vi "Orient Curves.vi"(8 "error in (no error)":errorcluster, 9 "Curve 2 In":cluster{"X":dbl, "Y":dbl}[](array[cluster]), 10 "Curve 1 In":cluster{"X":dbl, "Y":dbl}[](array[cluster]), 11 "Tool Funnel in":refnum<class "Tool Funnel.lvclass">) -> (0 "error out":errorcluster, 1 "Curve 2 Out":cluster{"X":dbl, "Y":dbl}[](array[cluster]), 2 "Curve 1 Out":cluster{"X":dbl, "Y":dbl}[](array[cluster]), 3 "Tool Funnel out":refnum<class "Tool Funnel.lvclass">)   [LabVIEW 2019, in "Tool Funnel.lvclass"]
uses:
  Tool Funnel.lvclass
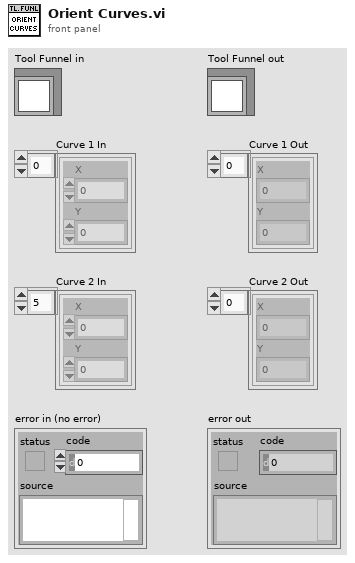
[diagram p1: front panel]
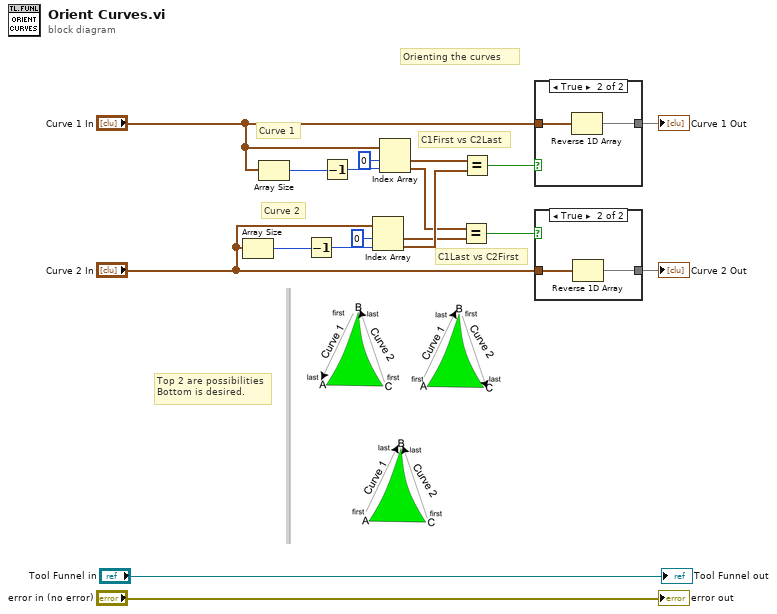
[diagram p0: block diagram]
diagram:
  # "Top 2 are possibilities\nBottom is desired."
  # "C1Last vs C2First"
  # "C1First vs C2Last"
  # "Orienting the curves"
  # "Curve 2"
  # "Curve 1"
  n1 = Array Size(array="Curve 2 In") -> (size(s)=w16:i32)
  n2 = Array Size(array="Curve 1 In") -> (size(s)=w12:i32)
  n3 = Decrement(x=w16) -> (x-1=w14:i32)
  n4 = Decrement(x=w12) -> (x-1=w11:i32)
  n5 = Index Array(array="Curve 2 In", index #1=0 ("index"), index #2=w14) -> (element #1=w6:cluster{"X":dbl, "Y":dbl}, element #2=w7:cluster{"X":dbl, "Y":dbl})
  n6 = Index Array(array="Curve 1 In", index #1=0 ("index"), index #2=w11) -> (element #1=w10:cluster{"X":dbl, "Y":dbl}, element #2=w5:cluster{"X":dbl, "Y":dbl})
  n7 = Equal?(x=w5, y=w6) -> (x = y?=w8:bool)
  n8 = Equal?(x=w10, y=w7) -> (x = y?=w9:bool)
  n9 = case shown="True" w9 {
    tunnel: "Curve 1 In" -> [w19 w21]
    tunnel: [w19 w20] -> w2
    frame False {
    }
    frame True {
      n10 = Reverse 1D Array(array=w21) -> (reversed array=w20:cluster{"X":dbl, "Y":dbl}[])
    }
  }
  "Curve 1 Out" <- w2
  n11 = case shown="True" w8 {
    tunnel: "Curve 2 In" -> [w22 w24]
    tunnel: [w22 w23] -> w3
    frame False {
    }
    frame True {
      n12 = Reverse 1D Array(array=w24) -> (reversed array=w23:cluster{"X":dbl, "Y":dbl}[])
    }
  }
  "Curve 2 Out" <- w3
  "error out" <- "error in (no error)"
  "Tool Funnel out" <- "Tool Funnel in"
